vi "Sawtooth.vi"(6 "Reintalize?":bool, 8 "Voltage":dbl(knob) scale=0.0..5.0) -> (0 "Absolute Angle (rad)":dbl, 1 "Absolute Angle (deg)":dbl, 3 "Rotations":dbl)   [LabVIEW 2012]
doc: "Counts peaks and valleys in absolute encoder signal, and outputs the number of directed rotations performed."
panel:
  out "Waveform Chart":dbl(graph)
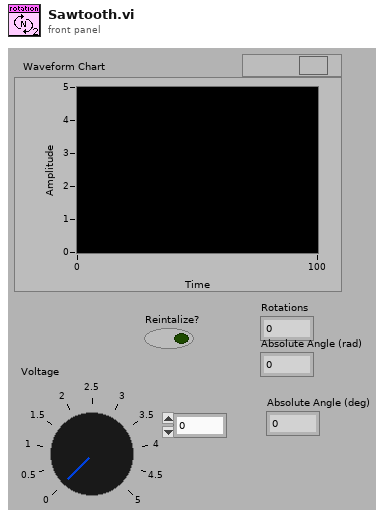
[diagram p1: front panel]
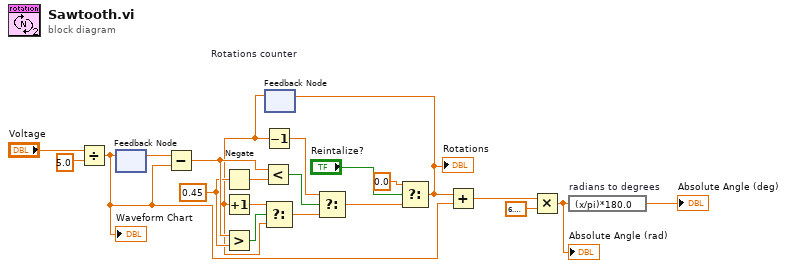
[diagram p0: block diagram]
diagram:
  w14 = 0.45 ("y")
  n1 = Divide(x="Voltage", y=5.0) -> (x/y=w5:dbl)
  "Waveform Chart" <- w5
  n2 = feedback #1() -> (w21:dbl)  [unwired: 1 out]
  n3 = feedback-in #1(w5) -> ()
  n4 = Subtract(x=w21, y=w5) -> (x-y=w20:dbl)
  n5 = Negate(x=w14) -> (-x=w13:dbl)
  n6 = Greater?(x=w20, y=w14) -> (0:w19:bool)
  n7 = Less?(x=w20, y=w13) -> (x < y?=w16:bool)
  n8 = feedback #2 "Rotations counter"() -> (w7:dbl)  [unwired: 1 in]
  n9 = Increment(x=w7) -> (x+1=w18:dbl)
  n10 = Decrement(x=w7) -> (x-1=w15:dbl)
  n11 = Select(t=w18, s=w19, f=w7) -> (s? t:f=w17:dbl)
  n12 = Select(t=w15, s=w16, f=w17) -> (s? t:f=w10:dbl)
  n13 = Select(t=0.0, s="Reintalize?", f=w10) -> (s? t:f=w6:dbl)
  "Rotations" <- w6
  n14 = feedback-in #2(w6) -> ()
  n15 = Add(x=w6, y=w5) -> (x+y=w4:dbl)
  n16 = Multiply(x=w4, y=6.283185307179586) -> (x*y=w2:dbl)
  "Absolute Angle (rad)" <- w2
  n17 = expression code="(x/pi)*180.0" "radians to degrees"(w2) -> (→"Absolute Angle (deg)":dbl)
